vi "依行或列索引2D数组(DBL)(冲突时的文件备份2013-05-03 10-46-30).vi"(8 "error in (no error)":errorcluster caption="错误输入（无错误）", 9 "选择行列":enum16{"行", "列"}(ring), 10 "索引":i32[](array[numeric]), 11 "输入数组":dbl[][](array[numeric])) -> (0 "error out":errorcluster caption="错误输出", 3 "元素":dbl[][](array[numeric]) format="%.2f")   [LabVIEW 2012]
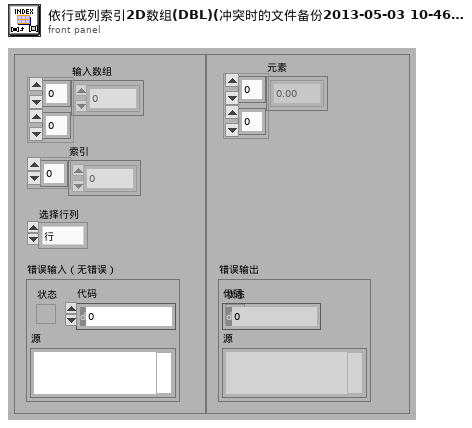
[diagram p1: front panel]
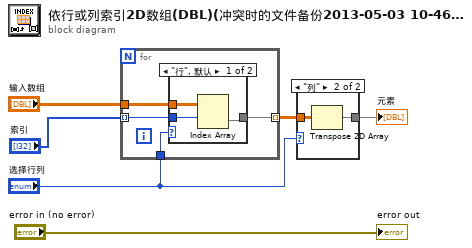
[diagram p0: block diagram]
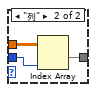
[diagram p3: hidden frame]
diagram:
  n1 = for {
    tunnel: "索引" -> [w8] mode=indexing
    tunnel: "输入数组" -> [w10]
    tunnel: [w9] -> w4 mode=indexing
    tunnel: "选择行列" -> [w7]
    n2 = case shown="\"行\", 默认" w7 {
      tunnel: w10 -> [w13 w16]
      tunnel: [w11 w15] -> w9
      tunnel: w8 -> [w12 w14]
      frame "行", Default {
        n3 = Index Array(array=w13, index (row)=w12) -> (element=w11:dbl[])  [unwired: 1 in]
      }
      frame "列" {
        n4 = Index Array(array=w16, index (col)=w14) -> (element=w15:dbl[])  [unwired: 1 in]
      }
    }
  }
  n5 = case shown="\"列\"" "选择行列" {
    tunnel: w4 -> [w17 w19]
    tunnel: [w17 w18] -> w3
    frame "行", Default {
    }
    frame "列" {
      n6 = Transpose 2D Array(2D array=w19) -> (transposed array=w18:dbl[][])
    }
  }
  "元素" <- w3
  "error out" <- "error in (no error)"
